vi "Close.vi"(8 "error in (no error)":errorcluster, 11 "Socket.UDP in":refnum<class "Socket.UDP.lvclass">) -> (0 "error out":errorcluster, 3 "Socket.UDP out":refnum<class "Socket.UDP.lvclass">)   [LabVIEW 2014, in "Socket.lvlib" / "Socket.UDP.lvclass"]
doc: "Closes an open connection."
uses:
  Socket.UDP.lvclass
  Socket.UDP.lvclass/Socket.UDP.ctl
  Socket.Base/Socket.Base.lvclass/Socket.Base.ctl
  Accessors/Read udp_refnum.vi
  Accessors/Write udp_refnum.vi
  Socket.Base/Accessors/Write connected.vi
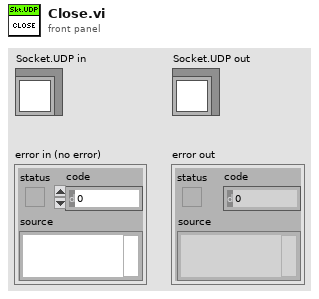
[diagram p1: front panel]
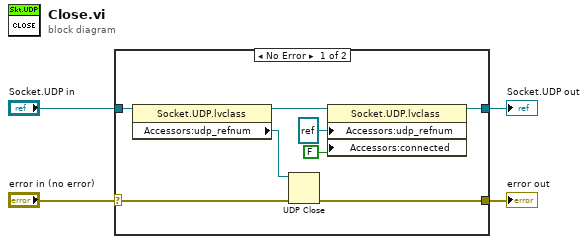
[diagram p0: block diagram]
diagram:
  n1 = case shown="No Error" "error in (no error)" {
    selector: "error in (no error)" -> [w11 w14]
    tunnel: [w8 w14] -> w3
    tunnel: [w9 w13] -> w1
    tunnel: "Socket.UDP in" -> [w12 w13]
    frame No Error {
      n2 = property class="Socket.UDP.lvclass"(reference=w12) -> (reference out=w10:refnum<class "Socket.UDP.lvclass">, "Accessors:udp_refnum"=w7:refnum<k16>)  [unwired: 1 in, 1 out]
      n3 = UDP Close(connection ID=w7, 8:w11) -> (error out=w8:errorcluster)  [unwired: 1 out]
      n4 = property class="Socket.UDP.lvclass"(reference=w10, "Accessors:udp_refnum"=refnum<k16> refnum ("udp_refnum"), "Accessors:connected"=FALSE ("connected")) -> (reference out=w9:refnum<class "Socket.UDP.lvclass">)  [unwired: 1 in, 1 out]
    }
    frame Error {
    }
  }
  "error out" <- w3
  "Socket.UDP out" <- w1
